vi "Destroy Parallel Events.vi"(8 "error in (no error)":errorcluster, 11 "CIFPluginManager in":refnum<class "CIFPluginManager.lvclass">) -> (0 "error out":errorcluster, 3 "CIFPluginManager out":refnum<class "CIFPluginManager.lvclass">)   [LabVIEW 2021, in "CIFPluginManager.lvclass"]
uses:
  CIFPluginManager.lvclass
  CIFPluginManager.lvclass/CIFPluginManager.ctl
  typedef/Parallel Events.ctl
  typedef/Loader Load Command.ctl
  Common/typedef/Loader Type.ctl
  typedef/Plugin Load Command.ctl
  typedef/Discover Command.ctl
  Common/Manager Common.lvlib
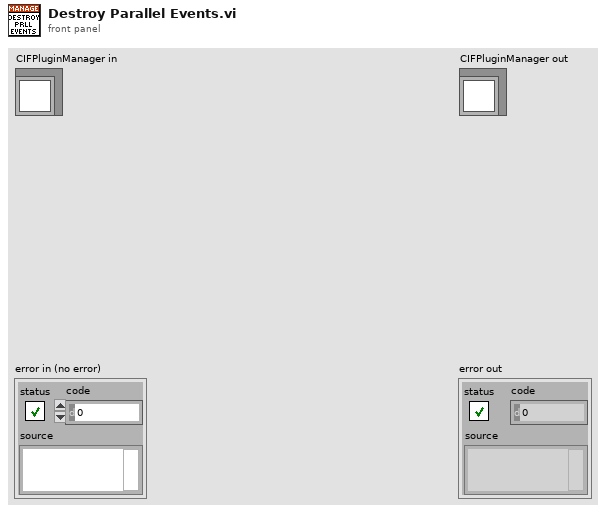
[diagram p1: front panel]
types:
  T1 = typedef "CIFPluginManager.lvclass/Parallel Events.ctl" = cluster{"Shutdown":refnum<user-event>, "Load Loader Events":refnum<user-event>, "Load Plugin Events":refnum<user-event>, "Trigger Discovery":refnum<user-event>, "Discover Events":refnum<user-event>, "Teardown":refnum<user-event>}
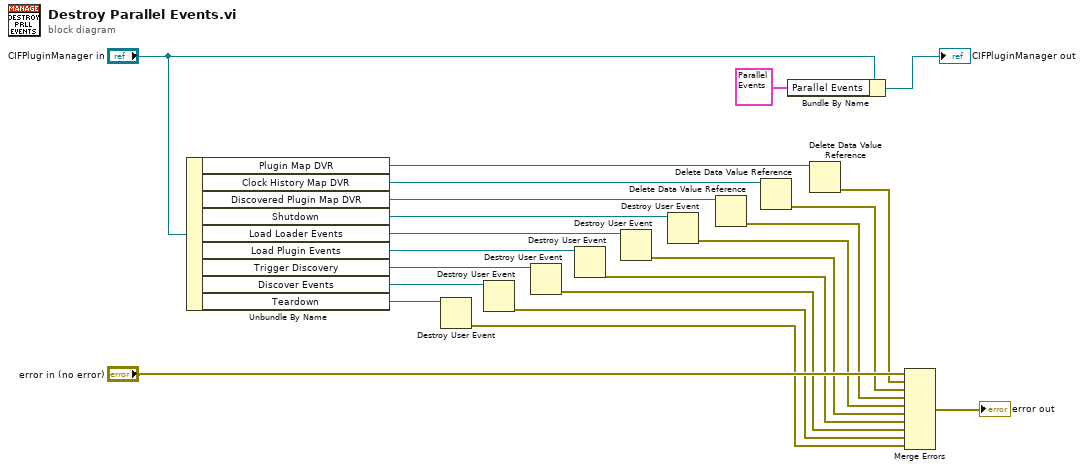
[diagram p0: block diagram]
diagram:
  n1 = Unbundle By Name("CIFPluginManager in") -> ("Plugin Map DVR"=w14:refnum<data-value>, "Clock History Map DVR"=w15:refnum<data-value>, "Discovered Plugin Map DVR"=w16:refnum<data-value>, "Shutdown"=w19:refnum<user-event>, "Load Loader Events"=w20:refnum<user-event>, "Load Plugin Events"=w8:refnum<user-event>, "Trigger Discovery"=w7:refnum<user-event>, "Discover Events"=w4:refnum<user-event>, "Teardown"=w2:refnum<user-event>)
  n2 = Destroy User Event(user event=w2) -> (error out=w1:errorcluster)  [unwired: 1 in]
  n3 = Destroy User Event(user event=w4) -> (error out=w3:errorcluster)  [unwired: 1 in]
  n4 = Destroy User Event(user event=w7) -> (error out=w5:errorcluster)  [unwired: 1 in]
  n5 = Destroy User Event(user event=w8) -> (error out=w6:errorcluster)  [unwired: 1 in]
  n6 = Destroy User Event(user event=w20) -> (error out=w9:errorcluster)  [unwired: 1 in]
  n7 = Destroy User Event(user event=w19) -> (error out=w10:errorcluster)  [unwired: 1 in]
  n8 = Delete Data Value Reference(data value reference=w16) -> (error out=w11:errorcluster)  [unwired: 1 in, 1 out]
  n9 = Delete Data Value Reference(data value reference=w15) -> (error out=w12:errorcluster)  [unwired: 1 in, 1 out]
  n10 = Bundle By Name(cluster="CIFPluginManager in", "Parallel Events"=T1 {"Shutdown"=refnum, "Load Loader Events"=refnum, "Load Plugin Events"=refnum, "Trigger Discovery"=refnum, "Discover Events"=refnum, "Teardown"=refnum} ("Discovery Events")) -> (→"CIFPluginManager out":refnum<class "CIFPluginManager.lvclass">)
  n11 = Delete Data Value Reference(data value reference=w14) -> (error out=w13:errorcluster)  [unwired: 1 in, 1 out]
  n12 = Merge Errors("error in (no error)", w13, w12, w11, w10, w9, w6, w5, w3, w1) -> (→"error out":errorcluster)
